vi "Cache.DUT.WriteComponent.vi"(6 "Time (now)":timestamp, 7 "Idx":i32, 8 "error in (no error)":errorcluster, 10 "ProdComp":T1) -> (0 "error out":errorcluster)   [LabVIEW 2016]
uses:
  Cache.ProductComponent.Data.ctl
  Global/ApplicationGlobal.vi
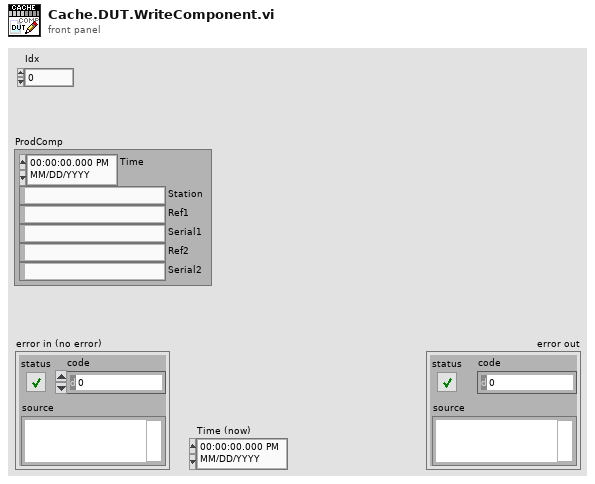
[diagram p1: front panel]
types:
  T1 = typedef "Cache.ProductComponent.Data.ctl" = cluster{"Time":timestamp, "Station":string, "Ref1":string, "Serial1":string, "Ref2":string, "Serial2":string}
  T2 = enum16{"open", "open or create", "create or replace", "create", "open (read-only)"}
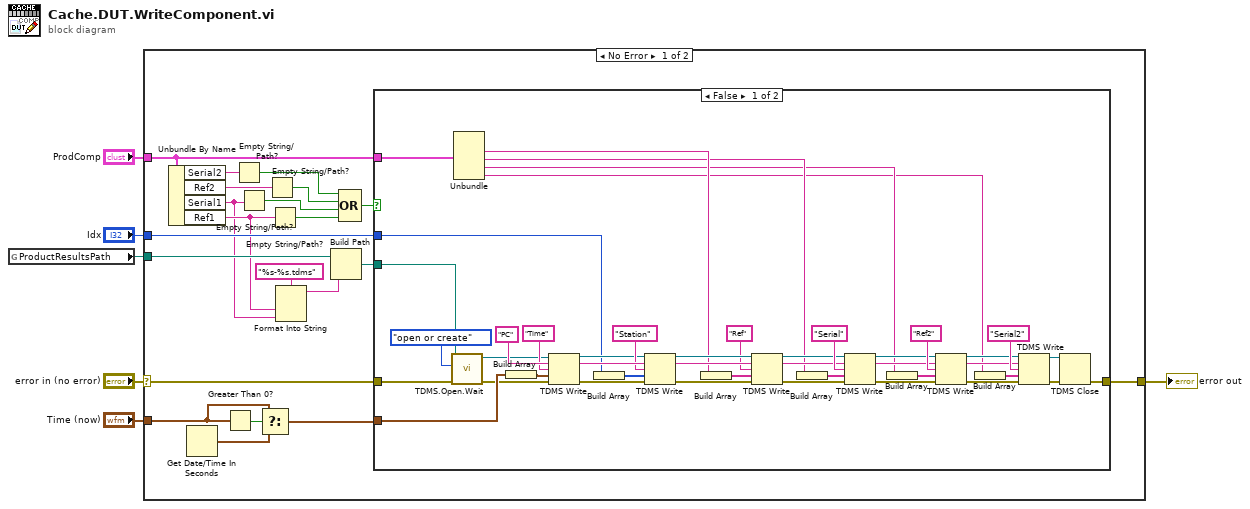
[diagram p0: block diagram]
diagram:
  n1 = global read "ApplicationGlobal.vi" "ProductResultsPath"() -> (w4:path)
  n2 = case shown="No Error" "error in (no error)" {
    selector: "error in (no error)" -> [w10 w72]
    tunnel: [w11 w72] -> w6
    tunnel: w4 -> [w27 _]
    tunnel: "ProdComp" -> [w19 _]
    tunnel: "Idx" -> [w13 _]
    tunnel: "Time (now)" -> [w15 _]
    frame No Error {
      n3 = Unbundle By Name(w19) -> ("Serial2"=w23:string, "Ref2"=w24:string, "Serial1"=w8:string, "Ref1"=w9:string)
      n4 = Get Date/Time In Seconds() -> (seconds since 1Jan1904=w17:timestamp)
      n5 = Greater Than 0?(x=w15) -> (x > 0?=w16:bool)
      n6 = Empty String/Path?(string/path=w23) -> (empty?=w18:bool)
      n7 = Empty String/Path?(string/path=w8) -> (empty?=w21:bool)
      n8 = Select(t=w15, s=w16, f=w17) -> (s? t:f=w14:timestamp)
      n9 = Empty String/Path?(string/path=w24) -> (empty?=w22:bool)
      n10 = Empty String/Path?(string/path=w9) -> (empty?=w20:bool)
      n11 = Format Into String(format string="%s-%s.tdms" ("pattern"), w9, w8) -> (resulting string=w26:string)  [unwired: 2 in, 1 out]
      n12 = Build Path(base path=w27, name or relative path=w26) -> (appended path=w7:path)
      n13 = Compound Arithmetic op=OR(w18, w22, w21, w20) -> (w12:bool)
      n14 = case shown="False" w12 {
        tunnel: w10 -> [w29 w71]
        tunnel: [w33 w71] -> w11
        tunnel: w19 -> [w70 _]
        tunnel: w14 -> [w37 _]
        tunnel: w13 -> [w38 _]
        tunnel: w7 -> [w28 _]
        frame False {
          n15 = call "TDMS.Open.Wait.vi"("error in (no error)"=w29, "operation (open read-only)"=T2."open or create" ("operation (0:open)"), "file path"=w28) -> ("error out"=w31:errorcluster, "tdms file out"=w32:refnum<k34>)  [unwired: 7 in]
          n16 = Unbundle(w70) -> ("Ref1"=w42:string, "Serial1"=w41:string, "Ref2"=w40:string, "Serial2"=w39:string)  [unwired: 2 out]
          n17 = Build Array(w37) -> (w56:timestamp[])
          n18 = TDMS Write(0:w32, 5:"PC" ("group name in (Untitled)"), 7:"Time", 9:w56, 11:w31) -> (4:w63:refnum<k34>, 6:w68:string, 15:w64:errorcluster)  [unwired: 1 in, 1 out]
          n19 = Build Array(w38) -> (w65:i32[])
          n20 = TDMS Write(0:w63, 5:w68, 7:"Station", 9:w65, 11:w64) -> (4:w67:refnum<k34>, 6:w69:string, 15:w36:errorcluster)  [unwired: 1 in, 1 out]
          n21 = Build Array(w42) -> (w43:string[])
          n22 = TDMS Write(0:w67, 5:w69, 7:"Ref", 9:w43, 11:w36) -> (4:w45:refnum<k34>, 6:w46:string, 15:w44:errorcluster)  [unwired: 1 in, 1 out]
          n23 = Build Array(w41) -> (w47:string[])
          n24 = TDMS Write(0:w45, 5:w46, 7:"Serial", 9:w47, 11:w44) -> (4:w51:refnum<k34>, 6:w50:string, 15:w49:errorcluster)  [unwired: 1 in, 1 out]
          n25 = Build Array(w40) -> (w48:string[])
          n26 = TDMS Write(0:w51, 5:w50, 7:"Ref2", 9:w48, 11:w49) -> (4:w55:refnum<k34>, 6:w58:string, 15:w54:errorcluster)  [unwired: 1 in, 1 out]
          n27 = Build Array(w39) -> (w60:string[])
          n28 = TDMS Write(0:w55, 5:w58, 7:"Serial2", 9:w60, 11:w54) -> (4:w35:refnum<k34>, 15:w34:errorcluster)  [unwired: 1 in, 2 out]
          n29 = TDMS Close(8:w34, 11:w35) -> (0:w33:errorcluster)  [unwired: 1 out]
        }
        frame True {
        }
      }
    }
    frame Error {
    }
  }
  "error out" <- w6
